vi "set up timing channels.vi"(6 "Display Names":string[](array[string]), 9 "Instance Identifier":string[](array[string]), 10 "PROTO detailed timing ADVTIMING=TRUE":bool, 11 "Standard Engine Configuration in":refnum<class "Standard Engine Configuration.lvclass">) -> (3 "Standard Engine Configuration out":refnum<class "Standard Engine Configuration.lvclass">)   [LabVIEW 2013, in "Standard Engine Configuration.lvclass"]
uses:
  Execution Engine/Configuration/Standard Engine Configuration.lvclass
  <vilib>/NI/Tag Bus Module Framework/channel/channel classification.ctl
  <vilib>/NI/Configuration Framework/serializable configuration/NISE_CEF_serializable configuration.lvclass/NISE_CEF_serializable configuration.ctl
  <vilib>/NI/Tag Bus/tag/Data Type.ctl
  <vilib>/NI/Tag Bus/tag/tag descriptor.lvclass
  <vilib>/Utility/LVClass/Get LV Class Name.vi
  <vilib>/NI/Configuration Framework/error generator/NISE_error generator.vi
  <vilib>/NI/Tag Bus Module Framework/channel/TBM channel.lvclass
  <vilib>/NI/Module Execution Interface/Engine Configuration/engine configuration.lvclass
  <vilib>/NI/Configuration Framework/serializable configuration/NISE_CEF_serializable configuration.lvclass
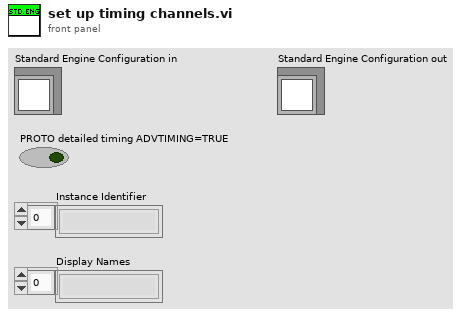
[diagram p1: front panel]
types:
  T1 = typedef "TBM channel.lvclass/channel classification.ctl" = enum16{"input data", "output data", "processing parameter", "processing result"}
  T2 = typedef "tag bus.lvlib/tag descriptor.lvclass/Data Type.ctl" = enum16{"Double", "Single", "I64", "I32", "I16", "I8", "U64", "U32", "U16", "U8", "Boolean", "String", "Array of Double", "Array of Single", "Array of I64", "Array of I32", "Array of I16", "Array of I8", "Array of U64", "Array of U32", "Array of U16", "Array of U8", "Array of Boolean", "Array of String"}
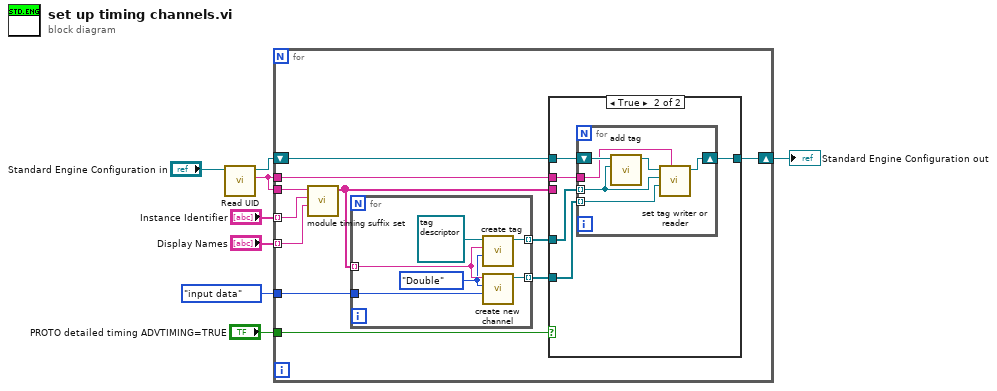
[diagram p0: block diagram]
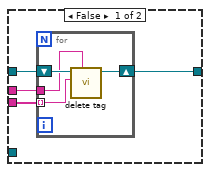
[diagram p2: hidden frame]
diagram:
  n1 = call <vilib>:"Read UID.vi"("configuration in"="Standard Engine Configuration in") -> ("instance id"=w8:string, "configuration out"=w4:refnum<class "Standard Engine Configuration.lvclass">)  [unwired: 8 in, 1 out]
  n2 = for {
    tunnel: "PROTO detailed timing ADVTIMING=TRUE" -> [w19]
    shift-right: [w17] -> w3
    shift-left: w4 -> [w18]
    tunnel: w8 -> [w16]
    tunnel: "Instance Identifier" -> [w15] mode=indexing
    tunnel: "Display Names" -> [w14] mode=indexing
    tunnel: channel_classification."input data" ("channel classification") -> [w12]
    tunnel: w8 -> [w10]
    n3 = call "module timing suffix set.vi"("mod alias"=w14, "mod id"=w15, "eng id"=w16) -> ("names"=w9:string[])  [unwired: 8 in]
    n4 = for {
      tunnel: w9 -> [w24] mode=indexing
      tunnel: [w25] -> w13 mode=indexing
      tunnel: w12 -> [w22]
      tunnel: [w21] -> w11 mode=indexing
      w23 = Data_Type."Double" ("data type")
      n5 = call-dynamic "create tag.vi"("data type"=w23, "name"=w24, "tag descriptor in"=refnum<class "tag descriptor.lvclass"> refnum) -> ("tag descriptor out"=w25:refnum<class "tag descriptor.lvclass">)  [unwired: 7 in, 1 out]
      n6 = call <vilib>:"create new channel.vi"("channel classification"=w22, "data type"=w23, "channel name"=w24) -> ("channel"=w21:refnum<class "TBM channel.lvclass">)  [unwired: 8 in]
    }
    n7 = case shown="True" w19 {
      tunnel: w18 -> [w29 w37]
      tunnel: [w27 w38] -> w17
      tunnel: w13 -> [_ w36]
      tunnel: w11 -> [_ w34]
      tunnel: w10 -> [w28 w35]
      tunnel: w9 -> [w26 _]
      frame False {
        n8 = for {
          tunnel: w28 -> [w32]
          shift-right: [w31] -> w27
          shift-left: w29 -> [w33]
          tunnel: w26 -> [w30] mode=indexing
          n9 = call <vilib>:"delete tag.vi"("owner ID"=w32, "tag name"=w30, "engine configuration in"=w33) -> ("engine configuration out"=w31:refnum<class "Standard Engine Configuration.lvclass">)  [unwired: 7 in, 1 out]
        }
      }
      frame True {
        n10 = for {
          shift-right: [w42] -> w38
          shift-left: w37 -> [w44]
          tunnel: w36 -> [w41] mode=indexing
          tunnel: w35 -> [w39]
          tunnel: w34 -> [w40] mode=indexing
          n11 = call <vilib>:"add tag.vi"("tag descriptor"=w41, "engine configuration in"=w44) -> ("engine configuration out"=w43:refnum<class "Standard Engine Configuration.lvclass">)  [unwired: 8 in, 1 out]
          n12 = call <vilib>:"set tag writer or reader.vi"("module GUID"=w39, "channel"=w40, "tag descriptor"=w41, "engine configuration in"=w43) -> ("engine configuration out"=w42:refnum<class "Standard Engine Configuration.lvclass">)  [unwired: 6 in, 1 out]
        }
      }
    }
  }
  "Standard Engine Configuration out" <- w3
